vi "pf_Init_Camera.vi"(7 "Interface Name":string, 8 "error in (no error)":errorcluster, 11 "IMAQ Session in":refnum<k11>) -> (0 "error out":errorcluster, 3 "IMAQ Session out":refnum<k11>)   [LabVIEW 2025, in "Photonfocus_Toolkit.lvlib"]
uses:
  Photonfocus_Toolkit.lvlib
  _Private/Controls/pf_Camera_Control.ctl
  _Private/Controls/pf_PeakDetector_Mode.ctl
  _Private/Controls/pf_Camera_ctrl_mngr_action.ctl
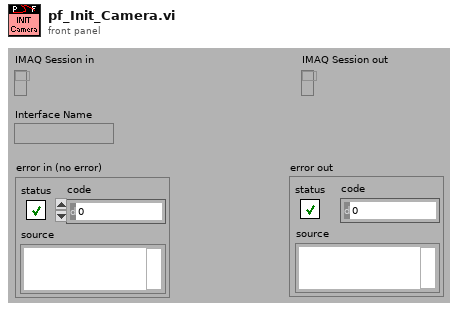
[diagram p1: front panel]
types:
  T1 = typedef "Photonfocus_Toolkit.lvlib/pf_Camera_ctrl_mngr_action.ctl" = enum16{"Create", "Destroy", "Set", "Get"}
  T2 = typedef "Photonfocus_Toolkit.lvlib/pf_Camera_Control.ctl" = cluster{"Port Name":string, "Port Number":i32, "IMAQ Session":refnum<k11>, "PeakDetector_Mode":T3, "Window.W":u32, "Window.H":u32}
  T3 = typedef "Photonfocus_Toolkit.lvlib/pf_PeakDetector_Mode.ctl" = enum16{"Undefined", "2D only", "2D and 3D", "3D only"}
  T4 = typedef "Photonfocus_Toolkit.lvlib/pf_Port_Info.ctl" = cluster{"Port Number":i32, "Manufacturer Name":string, "Port Name":string, "CLALLSERIAL Version":T5, "Port Type":T6}
  T5 = typedef "Photonfocus_Toolkit.lvlib/pf_CLALLSERIAL_Version.ctl" = enum16{"Undefined", "No CLALLSERIAL port", "CL_DLL_VERSION_NO_VERSION", "CL_DLL_VERSION_1_0", "CL_DLL_VERSION_1_1"}
  T6 = typedef "Photonfocus_Toolkit.lvlib/pf_Port_Type.ctl" = enum16{"Undefined", "CLALLSERIAL port", "port with clser.dll", "USB port", "RS-232 port"}
  T7 = typedef "Photonfocus_Toolkit.lvlib/pf_Property_Cluster.ctl" = cluster{"Name":string, "Type":T8, "Float.Min":sgl, "Float.Max":sgl, "Float.Value":sgl, "Int.Min":u32, "Int.Max":u32, "Int.Value":u32, "String.Value":string, "MODE.Values":string[], "MODE.Index":i32, "Flag":T9}
  T8 = typedef "Photonfocus_Toolkit.lvlib/pf_Property_Type.ctl" = enum16{"Undefined", "PF_ROOT", "PF_INT", "PF_FLOAT", "PF_BOOL", "PF_MODE", "PF_REGISTER", "PF_STRING", "PF_BUFFER", "PF_STRUCT", "PF_ARRAY", "PF_COMMAND", "PF_EVENT"}
  T9 = typedef "Photonfocus_Toolkit.lvlib/pf_Property_Flag.ctl" = enum16{"Undefined", "RO", "WO", "RW"}
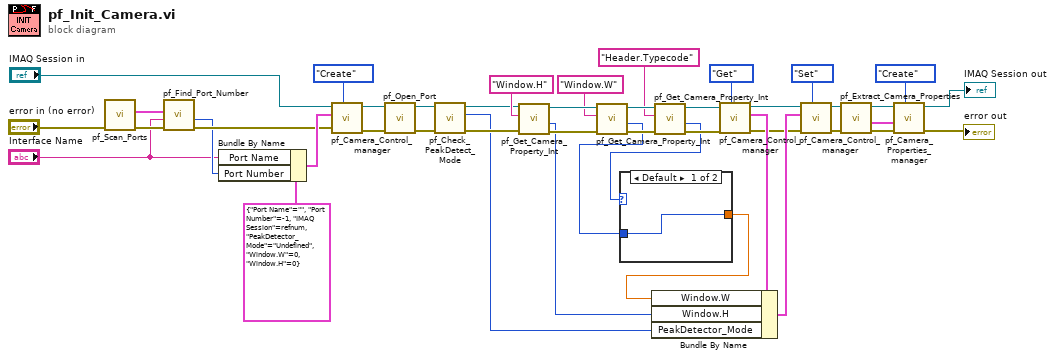
[diagram p0: block diagram]
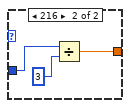
[diagram p2: hidden frame]
diagram:
  n1 = call "pf_Scan_Ports.vi"("error in (no error)"="error in (no error)") -> ("error out"=w40:errorcluster, "Ports Info Array"=w38:T4[])  [unwired: 9 out]
  n2 = call "pf_Find_Port_Number.vi"("error in (no error)"=w40, "Port Name"="Interface Name", "Port Info array"=w38) -> ("error out"=w39:errorcluster, "Port Number found"=w37:i32)  [unwired: 1 in, 6 out]
  n3 = Bundle By Name(cluster=T2 {"Port Name"="", "Port Number"=-1, "IMAQ Session"=refnum, "PeakDetector_Mode"=enum."Undefined", "Window.W"=0, "Window.H"=0} ("Camera Control in"), "Port Name"="Interface Name", "Port Number"=w37) -> (w42:T2)
  n4 = call "pf_Camera_Control_manager.vi"("Action"=pf_Camera_ctrl_mngr_action."Create", "error in (no error)"=w39, "Camera Control in"=w42, "IMAQ Session in"="IMAQ Session in") -> ("error out"=w35:errorcluster, "IMAQ Session out"=w36:refnum<k11>)  [unwired: 6 out]
  n5 = call "pf_Open_Port.vi"("error in (no error)"=w35, "IMAQ Session in"=w36) -> ("error out"=w13:errorcluster, "IMAQ Session out"=w12:refnum<k11>)  [unwired: 8 out]
  n6 = call "pf_Check_PeakDetect_Mode.vi"("error in"=w13, "IMAQ Session in"=w12) -> ("error out"=w10:errorcluster, "PeakDetector_Mode"=w9:T3, "IMAQ Session out"=w11:refnum<k11>)  [unwired: 7 out]
  n7 = call "pf_Get_Camera_Property_Int.vi"("error in (no error)"=w10, "Property Name"="Window.H" ("pProperty"), "IMAQ Session in"=w11) -> ("error out"=w21:errorcluster, "Property Value"=w17:i32, "IMAQ Session out"=w19:refnum<k11>)  [unwired: 6 out]
  n8 = call "pf_Get_Camera_Property_Int.vi"("error in (no error)"=w21, "Property Name"="Window.W" ("pProperty"), "IMAQ Session in"=w19) -> ("error out"=w6:errorcluster, "Property Value"=w2:i32, "IMAQ Session out"=w8:refnum<k11>)  [unwired: 6 out]
  n9 = call "pf_Get_Camera_Property_Int.vi"("error in (no error)"=w6, "Property Name"="Header.Typecode" ("pProperty"), "IMAQ Session in"=w8) -> ("error out"=w5:errorcluster, "Property Value"=w3:i32, "IMAQ Session out"=w7:refnum<k11>)  [unwired: 6 out]
  n10 = case shown="Default" w3 {
    tunnel: w2 -> [w45 w48]
    tunnel: [w45 w46] -> w1
    frame Default {
    }
    frame 216 {
      n11 = Divide(x=w48, y=3) -> (x/y=w46:dbl)
    }
  }
  n12 = call "pf_Camera_Control_manager.vi"("Action"=pf_Camera_ctrl_mngr_action."Get", "error in (no error)"=w5, "IMAQ Session in"=w7) -> ("error out"=w24:errorcluster, "Camera Control out"=w27:T2, "IMAQ Session out"=w25:refnum<k11>)  [unwired: 1 in, 5 out]
  n13 = Bundle By Name(cluster=w27, "Window.W"=w1, "Window.H"=w17, "PeakDetector_Mode"=w9) -> (w26:T2)
  n14 = call "pf_Camera_Control_manager.vi"("Action"=pf_Camera_ctrl_mngr_action."Set", "error in (no error)"=w24, "Camera Control in"=w26, "IMAQ Session in"=w25) -> ("error out"=w23:errorcluster, "IMAQ Session out"=w22:refnum<k11>)  [unwired: 6 out]
  n15 = call "pf_Extract_Camera_Properties.vi"("error in (no error)"=w23, "IMAQ Session in"=w22) -> ("error out"=w34:errorcluster, "Properties Array"=w31:T7[], "IMAQ Session out"=w33:refnum<k11>)  [unwired: 7 out]
  n16 = call "pf_Camera_Properties_manager.vi"("Action"=pf_Camera_ctrl_mngr_action."Create", "error in (no error)"=w34, "Properties Array"=w31, "IMAQ Session in"=w33) -> ("error out"=→"error out":errorcluster, "IMAQ Session out"=→"IMAQ Session out":refnum<k11>)  [unwired: 1 in, 5 out]
